vi "HDPE Process and add Images.vi"(8 "error in (no error)":errorcluster, 9 "Process Image":T1, 10 "Color range array":T2[](array[typedef]) {"Color Mode" items=["RGB", "HSL", "HSV", "HSI"]}, 11 "Original Image":T1) -> (0 "error out":errorcluster, 3 "Image Dst Out":T1)   [LabVIEW 2019]
uses:
  <vilib>/vision/Image Controls.llb/IMAQ Image.ctl
  Controls/Color Range cluster.ctl
  <vilib>/vision/NI_Vision_Development_Module.lvlib
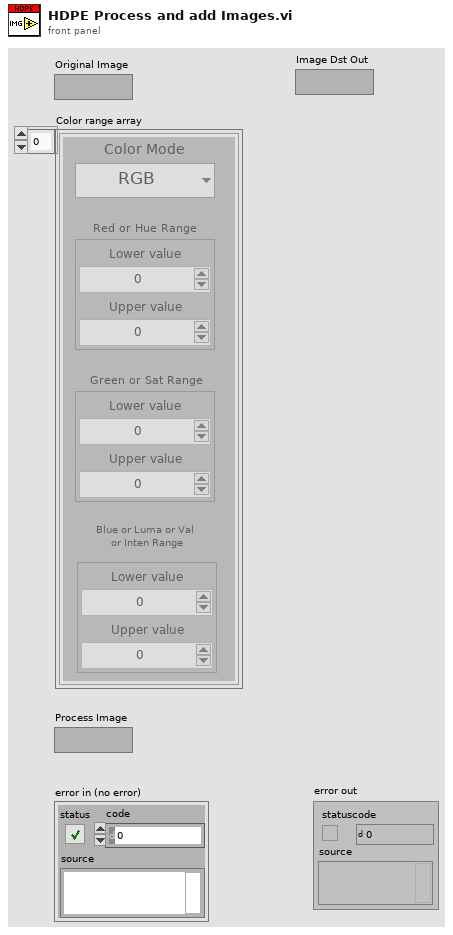
[diagram p1: front panel]
types:
  T1 = typedef "IMAQ Image.ctl" = refnum<image>
  T2 = typedef "Color Range cluster.ctl" = cluster{"Color Mode ":u16, "Red or Hue Range":cluster{"Lower value":i32, "Upper value":i32}, "Green or Sat Range":cluster{"Lower value":i32, "Upper value":i32}, "Blue or Luma or Val \nor Inten Range":cluster{"Lower value":i32, "Upper value":i32}}
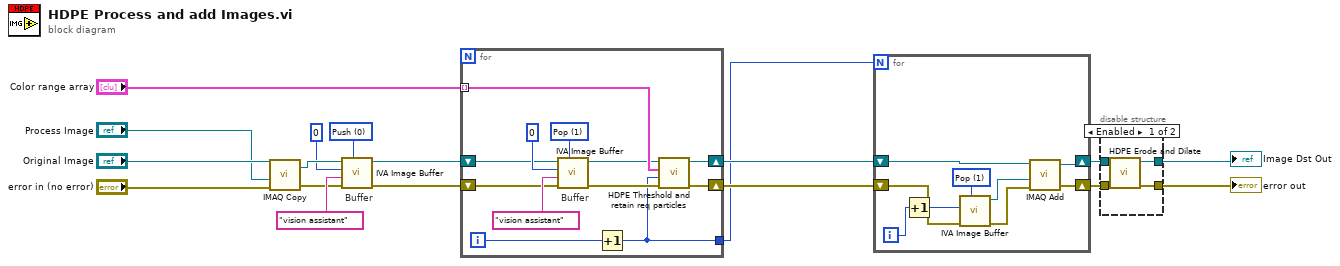
[diagram p0: block diagram]
diagram:
  w7 = u16 0 items=["Push", "Pop", "Reset"] ("Function")
  # "Buffer"
  n1 = call "IMAQ Copy"("error in (no error)"="error in (no error)", "Image Dst"="Process Image", "Image Src"="Original Image") -> ("error out"=w3:errorcluster, "Image Dst Out"=w8:T1)  [unwired: 3 in]
  n2 = call <vilib>:"IVA Image Buffer.vi"("Function"=w7, "error in (no error)"=w3, "Prefix"="vision assistant", "Buffer #"=0, "Image In"=w8) -> ("error out"=w10:errorcluster, "Image Out"=w11:T1)  [unwired: 5 out]
  n3 = for {
    shift-right: [w30] -> w16
    shift-left: w10 -> [w24]
    tunnel: "Color range array" -> [w29] mode=indexing
    shift-right: [w20] -> w15
    shift-left: w11 -> [w23]
    tunnel: [w19] -> w14
    i -> [w28]
    w27 = u16 1 items=["Push", "Pop", "Reset"] ("Function")
    # "Buffer"
    n4 = call <vilib>:"IVA Image Buffer.vi"("Function"=w27, "error in (no error)"=w24, "Prefix"="vision assistant", "Buffer #"=0, "Image In"=w23) -> ("error out"=w22:errorcluster, "Image Out"=w21:T1)  [unwired: 5 out]
    n5 = Increment(x=w28) -> (x+1=w19:i32)
    n6 = call "HDPE Threshold and retain req particles.vi"("error in (no error)"=w22, "Buffer"=w19, "Color ranges"=w29, "Refnum in"=w21) -> ("error out"=w30:errorcluster, "Image Out"=w20:T1)  [unwired: 6 in]
  }
  n7 = for {
    N: w14 -> [_]
    shift-right: [w34] -> w18
    shift-left: w16 -> [w36]
    shift-right: [w35] -> w17
    shift-left: w15 -> [w33]
    i -> [w32]
    w37 = u16 1 items=["Push", "Pop", "Reset"] ("Function")
    n8 = Increment(x=w32) -> (x+1=w31:i32)
    n9 = call <vilib>:"IVA Image Buffer.vi"("Function"=w37, "error in (no error)"=w36, "Buffer #"=w31) -> ("error out"=w39:errorcluster, "Image Out"=w38:T1)  [unwired: 2 in, 5 out]
    n10 = call "IMAQ Add"("Image Src A"=w33, "Image Src B"=w38, "error in (no error)"=w39) -> ("Image Dst Out"=w35:T1, "error out"=w34:errorcluster)  [unwired: 2 in, 2 out]
  }
  n11 = disable-structure shown="Enabled" {
    disable-tunnel: w18 -> [w43 w44]
    disable-tunnel: w17 -> [w42 w45]
    disable-tunnel: [w41 w44] -> w2
    disable-tunnel: [w40 w45] -> w1
    frame Enabled {
      n12 = call "HDPE Erode and Dilate.vi"("error in (no error)"=w43, "Image Src"=w42) -> ("error out"=w41:errorcluster, "Image Dst Out"=w40:T1)  [unwired: 8 in]
    }
    frame Disabled {
    }
  }
  "error out" <- w2
  "Image Dst Out" <- w1
